vi "Image_RAW_Get_Imagedata.vi"(7 "Image Data Config":T1={"Lines of Image Data"=0, "Bytes per Even Line"=0, "Bytes per Odd Line"=0, "Image Data Type"=44, "Total Image Data Block Size"=0, "Image Data Block Offset"=0} {"Image Data Type" format="%x"}, 8 "error in (no error)":errorcluster, 11 "Frame (U8)":u8[](array[numeric])) -> (0 "error out":errorcluster, 2 "Image Data Payload":u8[](array[numeric]))   [LabVIEW 2020]
uses:
  ctl/Image_Data_Config.ctl
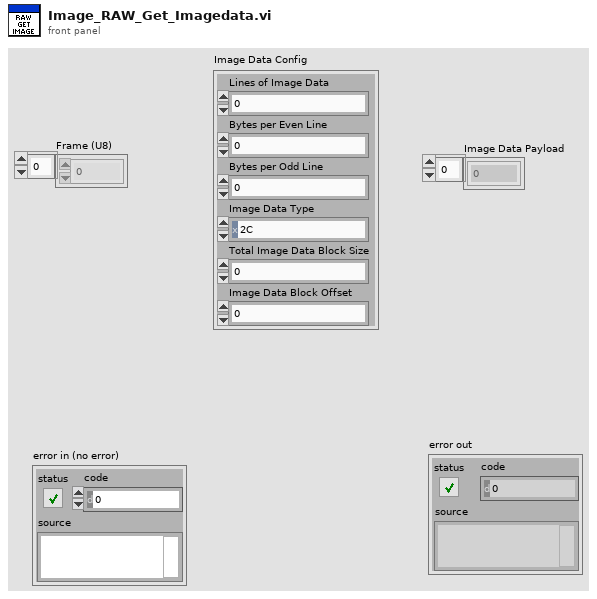
[diagram p1: front panel]
types:
  T1 = typedef "Image_Data_Config.ctl" = cluster{"Lines of Image Data":u16, "Bytes per Even Line":u16, "Bytes per Odd Line":u16, "Image Data Type":u8, "Total Image Data Block Size":u32, "Image Data Block Offset":u32}
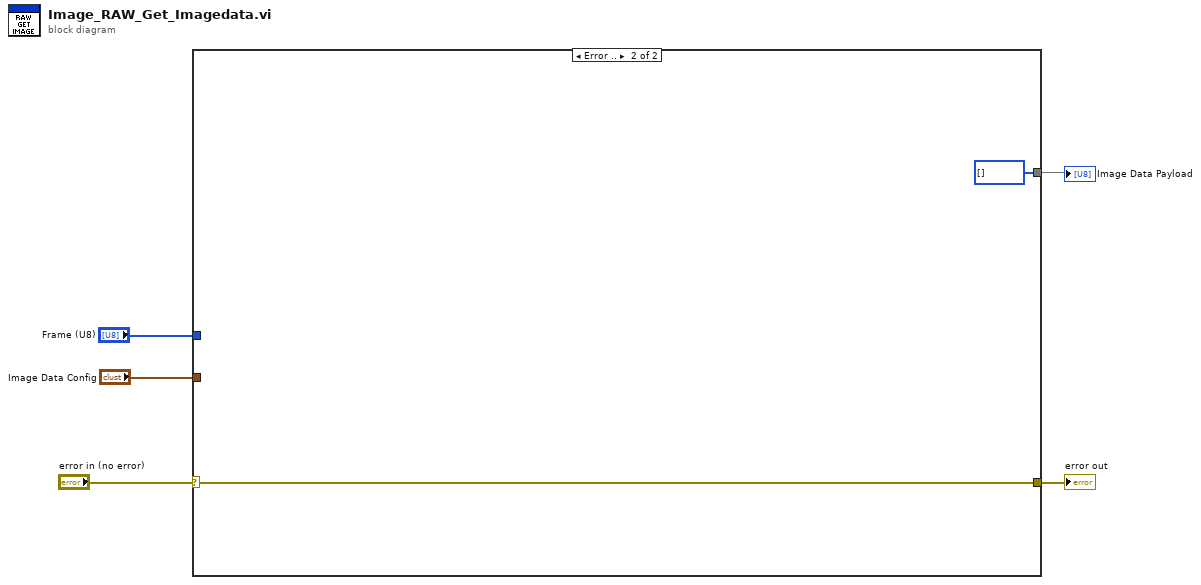
[diagram p0: block diagram]
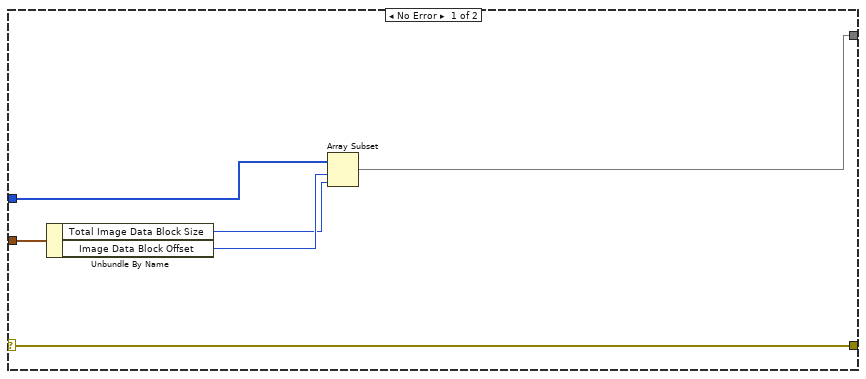
[diagram p2: hidden frame]
diagram:
  n1 = case shown="Error .." "error in (no error)" {
    selector: "error in (no error)" -> [w6 w13]
    tunnel: [w6 w13] -> w4
    tunnel: [w7 u8[] []] -> w3
    tunnel: "Image Data Config" -> [w11 _]
    tunnel: "Frame (U8)" -> [w10 _]
    frame No Error {
      n2 = Unbundle By Name(w11) -> ("Total Image Data Block Size"=w8:u32, "Image Data Block Offset"=w9:u32)
      n3 = Array Subset(array=w10, index=w9, length=w8) -> (w7:u8[])
    }
    frame Error {
    }
  }
  "error out" <- w4
  "Image Data Payload" <- w3
